vi "App Launcher.vi"() -> ()   [LabVIEW 2016]
uses:
  App/App/App.lvclass
  C:/Program Files/National Instruments/LabVIEW 2016/vi.lib/ActorFramework/Actor/Actor.lvclass
  <vilib>/ActorFramework/Actor/Actor.lvclass
panel:
  out "Error Out":errorcluster
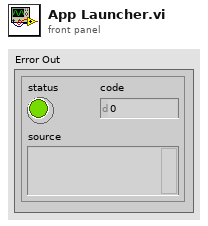
[diagram p1: front panel]
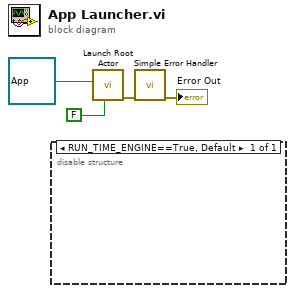
[diagram p0: block diagram]
diagram:
  n1 = disable-structure shown="RUN_TIME_ENGINE==True, Default" {
    frame condition #0 (active) {
    }
  }
  n2 = call <vilib>:"Launch Root Actor.vi"("Open Actor Core front panel? (F)"=FALSE, "Actor"=refnum<class "App.lvclass"> refnum ("App.lvlib:App.lvclass")) -> ("error out"=w2:errorcluster)  [unwired: 8 in, 1 out]
  n3 = call <vilib>:"Simple Error Handler.vi"("error in (no error)"=w2) -> ("error out"=→"Error Out":errorcluster)  [unwired: 4 in, 4 out]
